vi "Demo_Andon_logic_New.vi"(7 "Trigger":bool[](array[boolean]), 8 "IsActive?":bool, 9 "Inputs past":bool[](array[boolean]), 10 "Inputs":bool[](array[boolean]), 11 "Outputs past":bool[](array[boolean])) -> (1 "Inputs to save":bool[](array[boolean]), 2 "Outputs OUT":bool[](array[boolean]), 6 "Outputs to card":string[](array[string]))   [LabVIEW 2017]
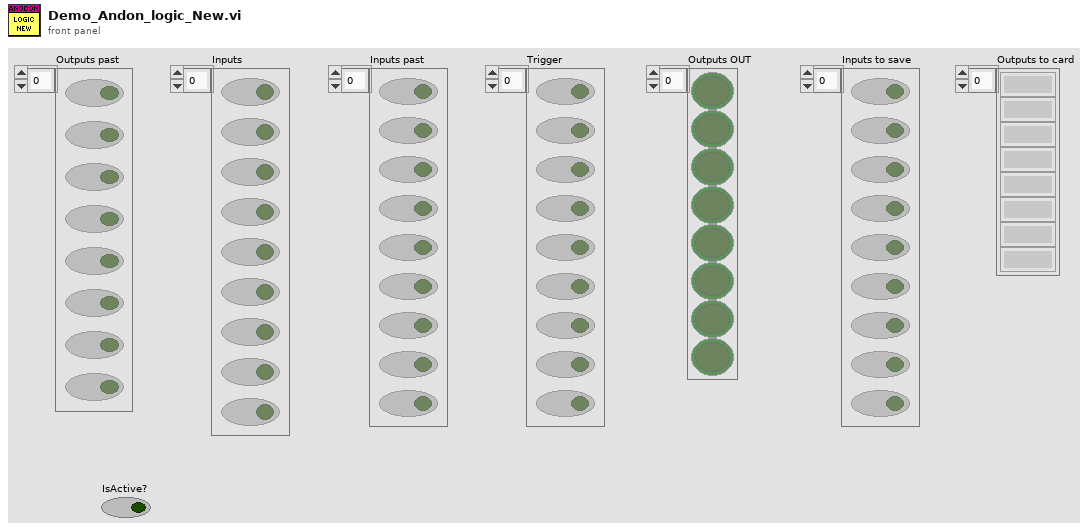
[diagram p1: front panel]
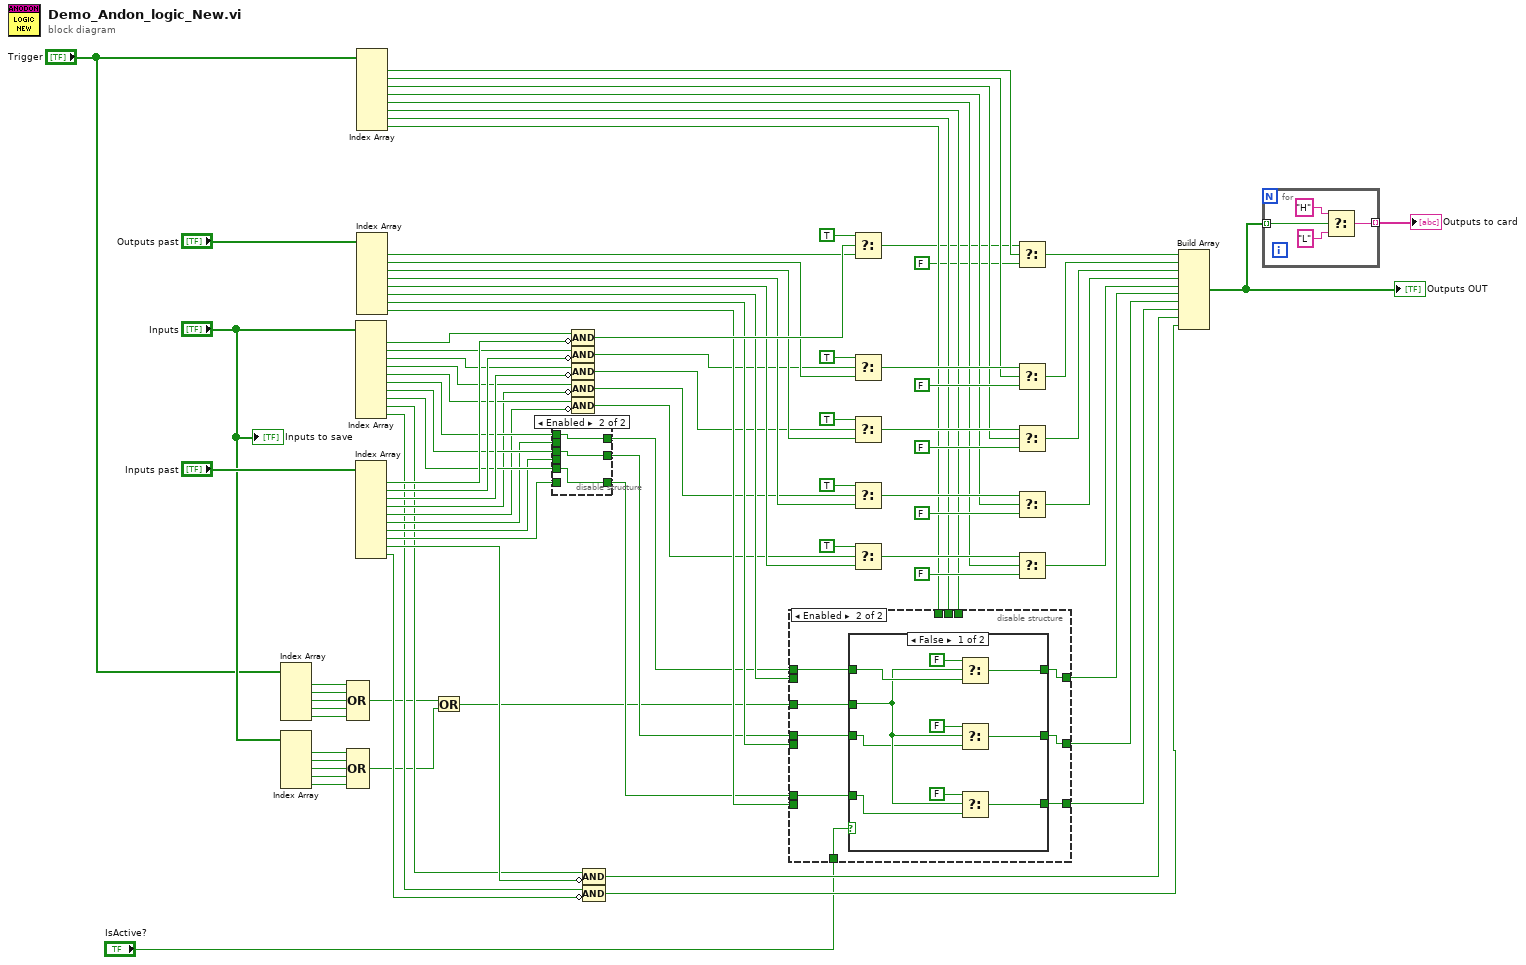
[diagram p0: block diagram]
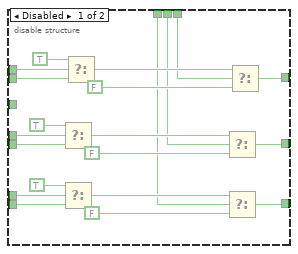
[diagram p2: hidden frame]
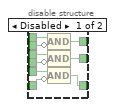
[diagram p4: hidden frame]
diagram:
  n1 = Index Array(array="Trigger") -> (element #1=w11:bool, element #2=w15:bool, element #3=w14:bool, element #4=w13:bool, element #5=w12:bool)  [unwired: 5 in]
  n2 = Index Array(array="Inputs") -> (element #1=w4:bool, element #2=w16:bool, element #3=w17:bool, element #4=w18:bool, element #5=w19:bool)  [unwired: 5 in]
  n3 = Compound Arithmetic op=OR(w11, w15, w14, w13, w12) -> (w9:bool)
  n4 = Compound Arithmetic op=OR(w4, w16, w17, w18, w19) -> (w8:bool)
  n5 = Index Array(array="Inputs") -> (element #1=w6:bool, element #2=w85:bool, element #3=w83:bool, element #4=w81:bool, element #5=w80:bool, element #6=w79:bool, element #7=w78:bool, element #8=w77:bool, element #9=w23:bool, element #10=w24:bool)  [unwired: 10 in]
  n6 = Index Array(array="Inputs past") -> (element #1=w86:bool, element #2=w84:bool, element #3=w82:bool, element #4=w76:bool, element #5=w75:bool, element #6=w74:bool, element #7=w73:bool, element #8=w72:bool, element #9=w25:bool, element #10=w26:bool)  [unwired: 10 in]
  n7 = Index Array(array="Trigger") -> (element #1=w69:bool, element #2=w33:bool, element #3=w32:bool, element #4=w31:bool, element #5=w30:bool, element #6=w29:bool, element #7=w28:bool, element #8=w27:bool)  [unwired: 8 in]
  n8 = Index Array(array="Outputs past") -> (element #1=w67:bool, element #2=w47:bool, element #3=w46:bool, element #4=w45:bool, element #5=w44:bool, element #6=w43:bool, element #7=w42:bool, element #8=w41:bool)  [unwired: 8 in]
  n9 = Or(x=w9, y=w8) -> (x .or. y?=w5:bool)
  n10 = disable-structure shown="Enabled" {
    disable-tunnel: w79 -> [w98 w101]
    disable-tunnel: w78 -> [w97 w100]
    disable-tunnel: w77 -> [w96 w99]
    disable-tunnel: w74 -> [w95 _]
    disable-tunnel: w73 -> [w94 _]
    disable-tunnel: w72 -> [w93 _]
    disable-tunnel: [w92 w99] -> w40
    disable-tunnel: [w91 w100] -> w39
    disable-tunnel: [w90 w101] -> w38
    frame Disabled {
      n11 = Compound Arithmetic op=AND(w98, invert w95) -> (w90:bool)
      n12 = Compound Arithmetic op=AND(w97, invert w94) -> (w91:bool)
      n13 = Compound Arithmetic op=AND(w96, invert w93) -> (w92:bool)
    }
    frame Enabled {
    }
  }
  n14 = Compound Arithmetic op=AND(w6, invert w86) -> (w70:bool)
  n15 = Compound Arithmetic op=AND(w85, invert w84) -> (w34:bool)
  n16 = Compound Arithmetic op=AND(w83, invert w82) -> (w35:bool)
  n17 = Compound Arithmetic op=AND(w81, invert w76) -> (w36:bool)
  n18 = Compound Arithmetic op=AND(w80, invert w75) -> (w37:bool)
  n19 = Compound Arithmetic op=AND(w23, invert w25) -> (w22:bool)
  n20 = Compound Arithmetic op=AND(w24, invert w26) -> (w21:bool)
  n21 = disable-structure shown="Enabled" {
    disable-tunnel: [w113 w129] -> w50
    disable-tunnel: [w112 w127] -> w49
    disable-tunnel: [w111 w125] -> w48
    disable-tunnel: w43 -> [w110 _]
    disable-tunnel: w42 -> [w109 _]
    disable-tunnel: w41 -> [w108 _]
    disable-tunnel: w40 -> [w107 w124]
    disable-tunnel: w39 -> [w106 w126]
    disable-tunnel: w38 -> [w105 w128]
    disable-tunnel: w29 -> [w104 _]
    disable-tunnel: w28 -> [w103 _]
    disable-tunnel: w27 -> [w102 _]
    disable-tunnel: "IsActive?" -> [_ w130]
    disable-tunnel: w5 -> [_ w123]
    frame Disabled {
      n22 = Select(t=TRUE ("f"), s=w106, f=w109) -> (s? t:f=w121:bool)
      n23 = Select(t=TRUE ("f"), s=w107, f=w108) -> (s? t:f=w115:bool)
      n24 = Select(t=TRUE ("f"), s=w105, f=w110) -> (s? t:f=w118:bool)
      n25 = Select(t=w121, s=w103, f=FALSE) -> (s? t:f=w112:bool)
      n26 = Select(t=w115, s=w102, f=FALSE) -> (s? t:f=w111:bool)
      n27 = Select(t=w118, s=w104, f=FALSE) -> (s? t:f=w113:bool)
    }
    frame Enabled {
      n28 = case shown="False" w130 {
        tunnel: [w138 w143] -> w129
        tunnel: w128 -> [w140 w143]
        tunnel: [w135 w142] -> w127
        tunnel: w126 -> [w133 w142]
        tunnel: [w131 w141] -> w125
        tunnel: w124 -> [w132 w141]
        tunnel: w123 -> [w134 _]
        frame False {
          n29 = Select(t=FALSE, s=w134, f=w140) -> (s? t:f=w138:bool)
          n30 = Select(t=FALSE, s=w134, f=w133) -> (s? t:f=w135:bool)
          n31 = Select(t=FALSE, s=w134, f=w132) -> (s? t:f=w131:bool)
        }
        frame True {
        }
      }
    }
  }
  n32 = Select(t=TRUE ("f"), s=w70, f=w67) -> (s? t:f=w2:bool)
  n33 = Select(t=TRUE ("f"), s=w34, f=w47) -> (s? t:f=w65:bool)
  n34 = Select(t=TRUE ("f"), s=w35, f=w46) -> (s? t:f=w62:bool)
  n35 = Select(t=TRUE ("f"), s=w36, f=w45) -> (s? t:f=w59:bool)
  n36 = Select(t=TRUE ("f"), s=w37, f=w44) -> (s? t:f=w56:bool)
  n37 = Select(t=w2, s=w69, f=FALSE) -> (s? t:f=w68:bool)
  n38 = Select(t=w65, s=w33, f=FALSE) -> (s? t:f=w54:bool)
  n39 = Select(t=w62, s=w32, f=FALSE) -> (s? t:f=w53:bool)
  n40 = Select(t=w59, s=w31, f=FALSE) -> (s? t:f=w52:bool)
  n41 = Select(t=w56, s=w30, f=FALSE) -> (s? t:f=w51:bool)
  n42 = Build Array(w68, w54, w53, w52, w51, w50, w49, w48, w22, w21) -> (w89:bool[])
  "Outputs OUT" <- w89
  n43 = for {
    tunnel: w89 -> [w145] mode=indexing
    tunnel: [w144] -> w88 mode=indexing
    n44 = Select(t="H", s=w145, f="L") -> (s? t:f=w144:string)
  }
  "Outputs to card" <- w88
  "Inputs to save" <- "Inputs"
